vi "Initialize From Settings.vi"(8 "error in (no error)":errorcluster, 10 "settings":cluster{"key":string, "value":string}[](array[cluster]), 11 "UDPlog Transfer Tx Configuration in":refnum<class "UDPlog Transfer Tx Configuration.lvclass">) -> (0 "error out":errorcluster, 3 "UDPlog Transfer Tx Configuration out":refnum<class "UDPlog Transfer Tx Configuration.lvclass">)   [LabVIEW 2023, in "UDPlog.lvlib" / "UDPlog Transfer Tx Configuration.lvclass"]
uses:
  UDPlog Transfer Tx Configuration.lvclass
  UDPlog Transfer Tx Configuration.lvclass/UDPlog Transfer Tx Configuration.ctl
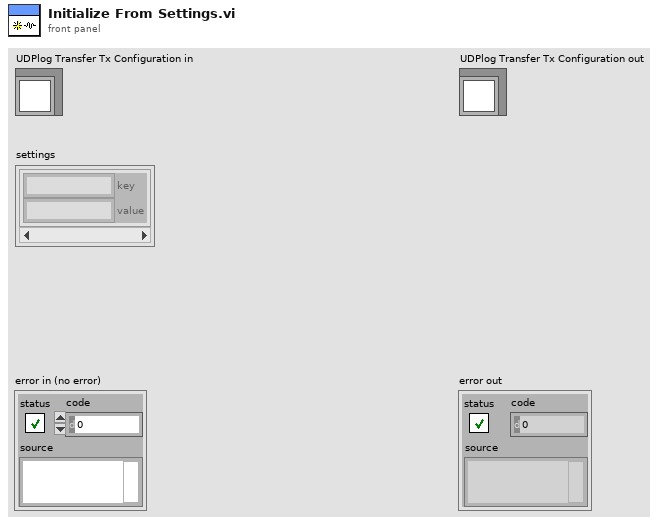
[diagram p1: front panel]
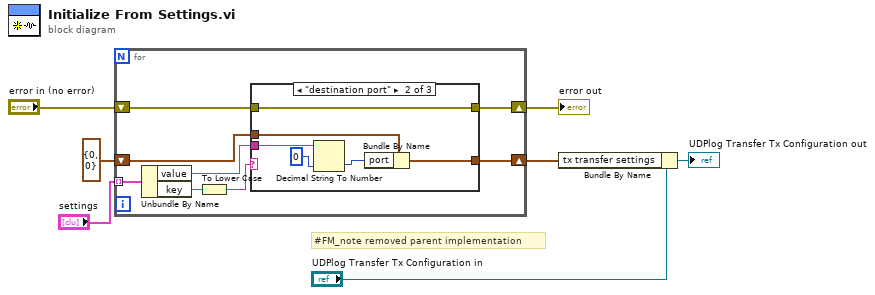
[diagram p0: block diagram]
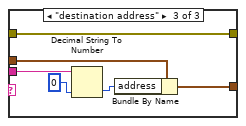
[diagram p3: hidden frame]
diagram:
  # "#FM_note removed parent implementation"
  n1 = for {
    shift-right: [w9] -> w1
    shift-left: "error in (no error)" -> [w14]
    shift-right: [w8] -> w2
    shift-left: cluster{"address":u32, "port":u16} {"address"=0, "port"=0} ("thread settings") -> [w11]
    tunnel: "settings" -> [w15] mode=indexing
    n2 = Unbundle By Name(w15) -> ("value"=w12:string, "key"=w13:string)
    n3 = To Lower Case(string=w13) -> (all lower case string=w10:string)
    n4 = case shown="\"destination port\"" w10 {
      tunnel: w14 -> [w16 w21 w27]
      tunnel: w12 -> [_ w20 w25]
      tunnel: w11 -> [w17 w23 w29]
      tunnel: [w17 w22 w28] -> w8
      tunnel: [w16 w21 w27] -> w9
      frame Default {
        # "Unknown Setting."
      }
      frame "destination port" {
        n5 = Decimal String To Number(string=w20, default (0L)=u16 0 ("default (0 I32)")) -> (number=w19:u16)  [unwired: 1 in, 1 out]
        n6 = Bundle By Name(cluster=w23, "port"=w19) -> (w22:cluster{"address":u32, "port":u16})
      }
      frame "destination address" {
        n7 = Decimal String To Number(string=w25, default (0L)=u32 0 ("default (0 I32)")) -> (number=w24:u32)  [unwired: 1 in, 1 out]
        n8 = Bundle By Name(cluster=w29, "address"=w24) -> (w28:cluster{"address":u32, "port":u16})
      }
    }
  }
  "error out" <- w1
  n9 = Bundle By Name(cluster="UDPlog Transfer Tx Configuration in", "tx transfer settings"=w2) -> (→"UDPlog Transfer Tx Configuration out":refnum<class "UDPlog Transfer Tx Configuration.lvclass">)
